vi "get_start_points.vi"(4 "error in":errorcluster, 7 "simx in":T2={"Config"={"Trajectory"={"Number of frames"=0, "Frame number"=0, "Trajectory"=""}, "Weather"={"id"=""}}, "Connections"={"Simulator Connection"=refnum, "server_ip"="127.0.0.1", "Port"=0, "Sensor connections"=[]}, "Map"={"lanes"={"x"=[], "y"=[], "z"=[]}, "StartPosition"={"start_points"={"locations"=[], "rotations"=[], "type"=[]}, "StartRotation"=[], "StartLocation"=[]}, "Draw Map Size"={"Width"=0, "Height"=0}, "DrawArea"={"min_Y"=0.0, "min_X"=0.0, "Scale X"=0.0, "Scale Y"=0.0}, "Map"=bytes[0], "Map Geojson"=""}}) -> (0 "error out":errorcluster, 2 "Starting Points":T1, 3 "simx out":T2={"Config"={"Trajectory"={"Number of frames"=0, "Frame number"=0, "Trajectory"=""}, "Weather"={"id"=""}}, "Connections"={"Simulator Connection"=refnum, "server_ip"="127.0.0.1", "Port"=0, "Sensor connections"=[]}, "Map"={"lanes"={"x"=[], "y"=[], "z"=[]}, "StartPosition"={"start_points"={"locations"=[], "rotations"=[], "type"=[]}, "StartRotation"=[], "StartLocation"=[]}, "Draw Map Size"={"Width"=0, "Height"=0}, "DrawArea"={"min_Y"=0.0, "min_X"=0.0, "Scale X"=0.0, "Scale Y"=0.0}, "Map"=bytes[0], "Map Geojson"=""}})   [LabVIEW 2025]
doc: "Send the GetStartPoints command to obtain the starting points for the map."
uses:
  controls/simx_connection.ctl
  controls/config.ctl
  controls/trajectory.ctl
  controls/weather.ctl
  controls/connections.ctl
  controls/start_points.ctl
  <vilib>/Utility/miscctls.llb/LVBoundsTypeDef.ctl
panel:
  out "status":bool
  out "response":string
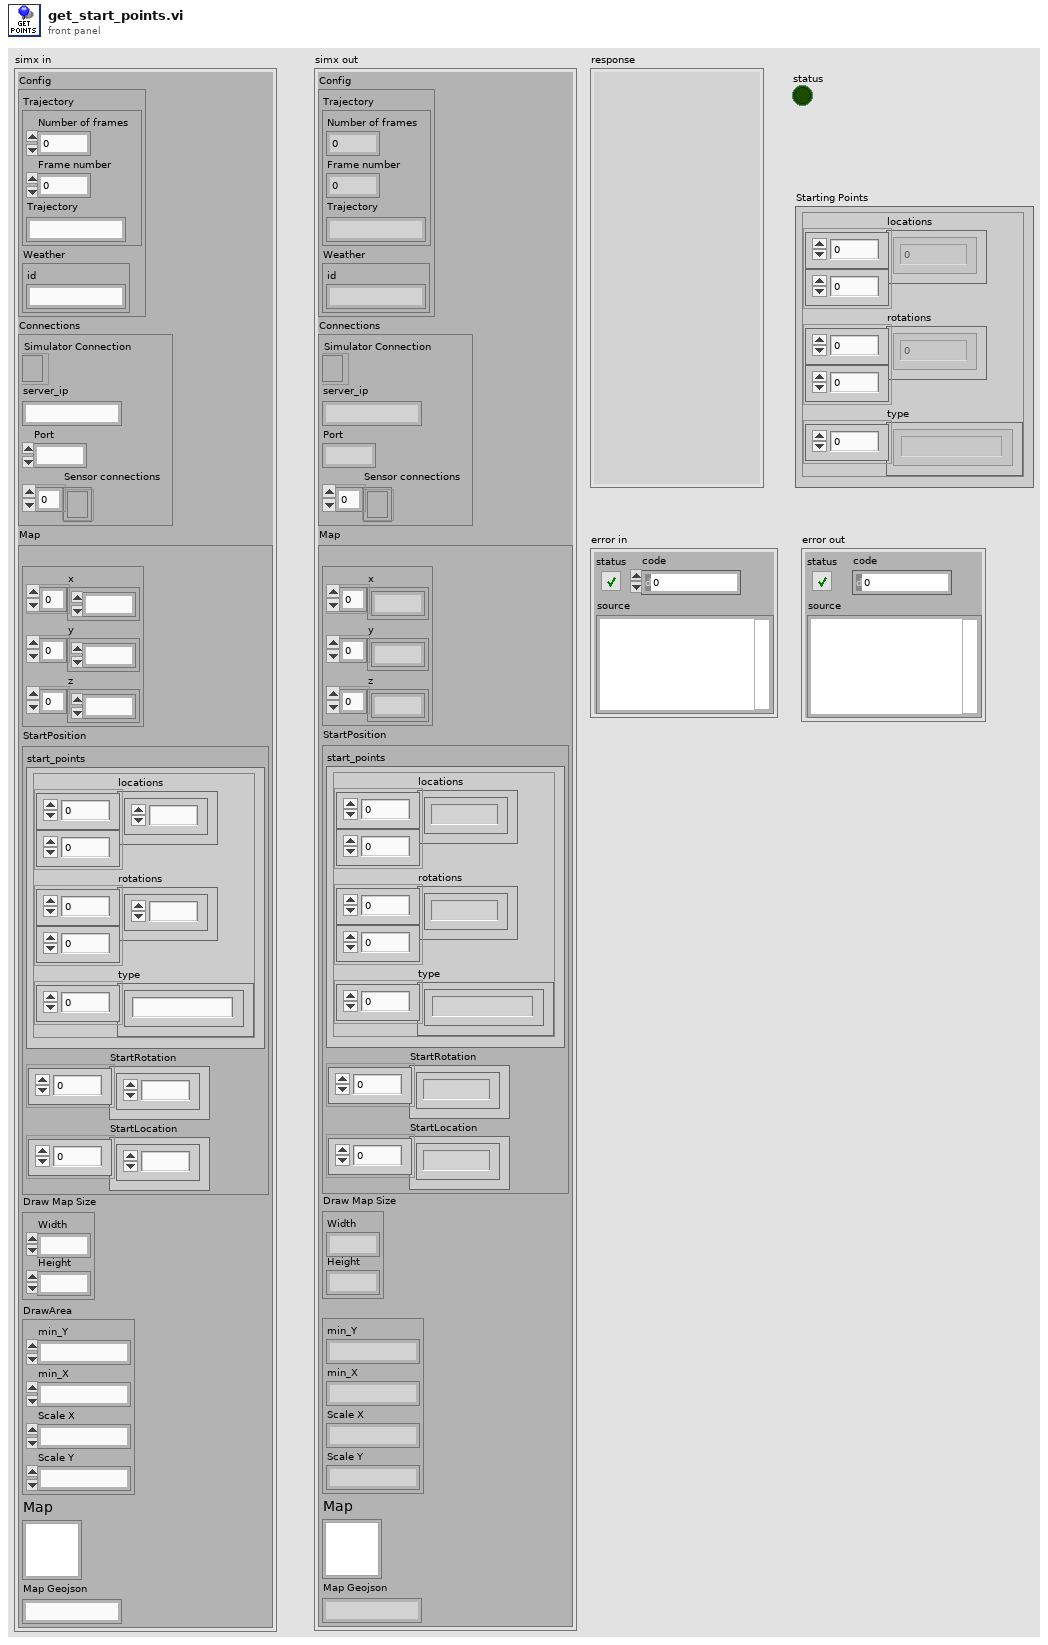
[diagram p1: front panel]
types:
  T1 = typedef "start_points.ctl" = cluster{"locations":dbl[][], "rotations":dbl[][], "type":string[]}
  T2 = typedef "simx_connection.ctl" = cluster{"Config":T3, "Connections":T6, "Map":cluster{"lanes":cluster{"x":dbl[], "y":dbl[], "z":dbl[]}, "StartPosition":cluster{"start_points":T1, "StartRotation":dbl[], "StartLocation":dbl[]}, "Draw Map Size":T7, "DrawArea":cluster{"min_Y":dbl, "min_X":dbl, "Scale X":dbl, "Scale Y":dbl}, "Map":picture, "Map Geojson":string}}
  T3 = typedef "config.ctl" = cluster{"Trajectory":T4, "Weather":T5}
  T4 = typedef "trajectory.ctl" = cluster{"Number of frames":i32, "Frame number":i32, "Trajectory":string}
  T5 = typedef "weather.ctl" = cluster{"id":string}
  T6 = typedef "connections.ctl" = cluster{"Simulator Connection":refnum<k5>, "server_ip":string, "Port":i32, "Sensor connections":refnum<k5>[]}
  T7 = typedef "LVBoundsTypeDef.ctl" = cluster{"Width":u32, "Height":u32}
  T8 = cluster{"locations":dbl[][], "rotations":dbl[][], "type":string[]}
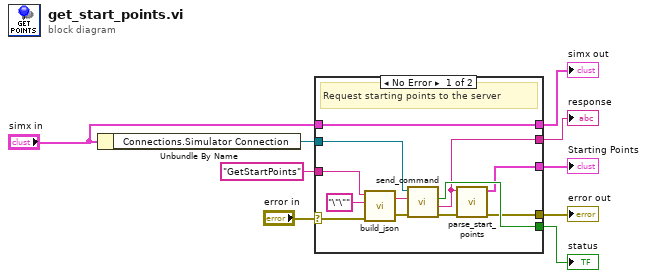
[diagram p0: block diagram]
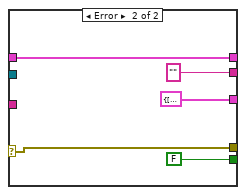
[diagram p2: hidden frame]
diagram:
  n1 = Unbundle By Name("simx in") -> ("Connections.Simulator Connection"=w2:refnum<k5>)
  n2 = case shown="No Error" "error in" {
    selector: "error in" -> [w17 w26]
    tunnel: [w11 w26] -> w9
    tunnel: [w15 "" ("response")] -> w8
    tunnel: [w21 FALSE ("success")] -> w5
    tunnel: "GetStartPoints" ("Command_ID") -> [w16 _]
    tunnel: "simx in" -> [w10 w23]
    tunnel: [w10 w23] -> w4
    tunnel: w2 -> [w18 _]
    tunnel: [w12 T8 {"locations"=[], "rotations"=[], "type"=[]} ("statt_locations")] -> w1
    frame No Error {
      # "Request starting points to the server"
      n3 = call "build_json.vi"("error in"=w17, "Message"="\"\"", "Command_ID"=w16) -> ("error out"=w19:errorcluster, "JSON Out"=w20:string)  [unwired: 1 in]
      n4 = call "send_command.vi"("error in"=w19, "JSON Command"=w20, "TCP Network Connection in"=w18) -> ("error out"=w14:errorcluster, "Response"=w15:string, "Success"=w21:bool)  [unwired: 1 in, 1 out]
      n5 = call "parse_start_points.vi"("error in"=w14, "Response"=w15) -> ("error out"=w11:errorcluster, "Start locations"=w12:T8)  [unwired: 4 in]
    }
    frame Error {
    }
  }
  "response" <- w8
  "error out" <- w9
  "status" <- w5
  "simx out" <- w4
  "Starting Points" <- w1
